vi "GetDatas.vi"(9 "电压传感器本地":dbl[](array[numeric]), 10 "电压传感器转换率":dbl[](array[numeric]), 11 "信号数据":dbl[][](array[numeric])) -> (3 "传感器信号":dbl[](array[numeric]))   [LabVIEW 2015, in "Logging.lvlib"]
uses:
  Logging.lvlib
  <vilib>/Analysis/baseanly.llb/Mean (DBL).vi
  <vilib>/Analysis/NI_AALBase.lvlib
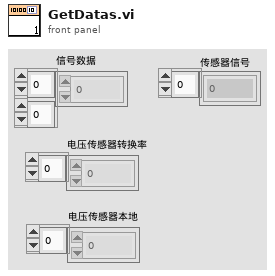
[diagram p1: front panel]
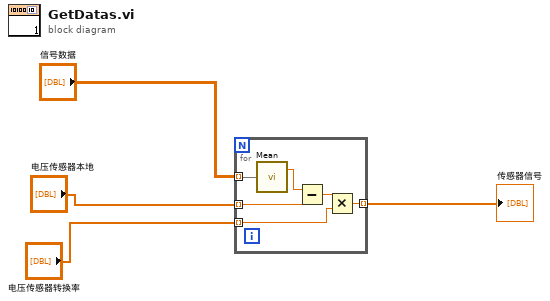
[diagram p0: block diagram]
diagram:
  n1 = for {
    tunnel: "信号数据" -> [w10] mode=indexing
    tunnel: "电压传感器本地" -> [w8] mode=indexing
    tunnel: "电压传感器转换率" -> [w6] mode=indexing
    tunnel: [w5] -> w3 mode=indexing
    n2 = call-poly <vilib>:"Mean.vi"("X"=w10) -> ("mean"=w9:dbl)  [unwired: 1 out]
    n3 = Subtract(x=w9, y=w8) -> (x-y=w7:dbl)
    n4 = Multiply(x=w7, y=w6) -> (x*y=w5:dbl)
  }
  "传感器信号" <- w3
